vi "AddSegment.vi"(8 "error in (no error)":errorcluster, 10 "point":cluster{"x":i16, "y":i16}, 11 "Line in":refnum<class "Line.lvclass">) -> (0 "error out":errorcluster, 3 "Line out":refnum<class "Line.lvclass">)   [LabVIEW 2014, in "Line.lvclass"]
uses:
  Line.lvclass
  Line.lvclass/Line.ctl
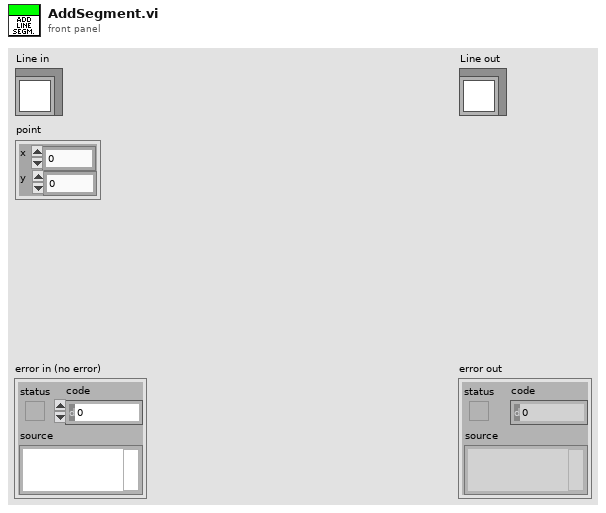
[diagram p1: front panel]
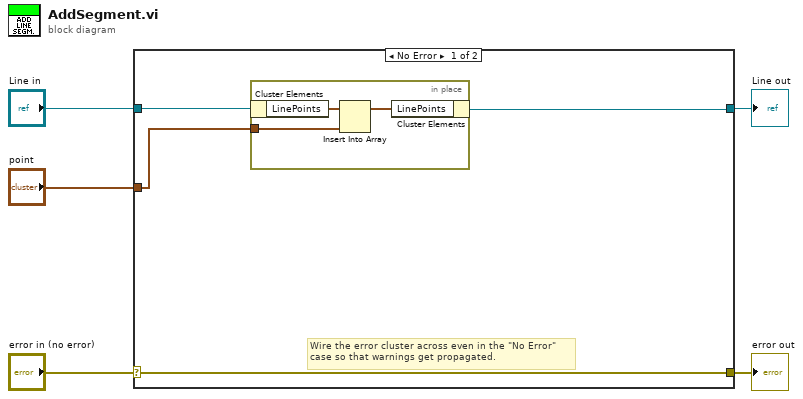
[diagram p0: block diagram]
diagram:
  n1 = case shown="No Error" "error in (no error)" {
    selector: "error in (no error)" -> [w9 w14]
    tunnel: [w9 w14] -> w4
    tunnel: [w6 w13] -> w2
    tunnel: "Line in" -> [w8 w13]
    tunnel: "point" -> [w7 _]
    frame No Error {
      # "Wire the error cluster across even in the \"No Error\"\ncase so that warnings get propagated."
      n2 = in-place {
        in-place-border: w7 -> [w12]
        n3 = in-place-cluster #1(w8) -> ("LinePoints"=w11:cluster{"x":i16, "y":i16}[])
        n4 = Insert Into Array(array=w11, new element=w12) -> (w10:cluster{"x":i16, "y":i16}[])  [unwired: 1 in]
        n5 = in-place-cluster #1("LinePoints"=w10) -> (w6:refnum<class "Line.lvclass">)
      }
    }
    frame Error {
    }
  }
  "error out" <- w4
  "Line out" <- w2
